vi "trunc_voltages.vi"(5 "Max":dbl, 7 "Min":dbl, 10 "transmissions[r=wl, c=v]":dbl[][](array[numeric]), 11 "voltages":dbl[](array[numeric])) -> (1 "trunc voltages":dbl[](array[numeric]), 2 "Min":dbl, 3 "Max":dbl, 4 "trunc transmissions[r=wl, c=v]":dbl[][](array[numeric]))   [LabVIEW 2019]
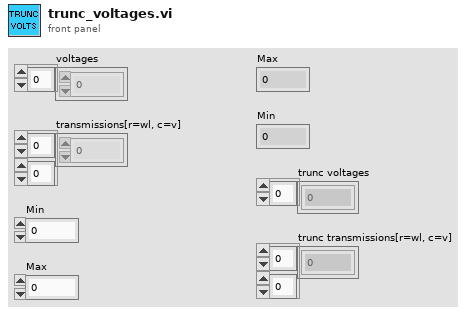
[diagram p1: front panel]
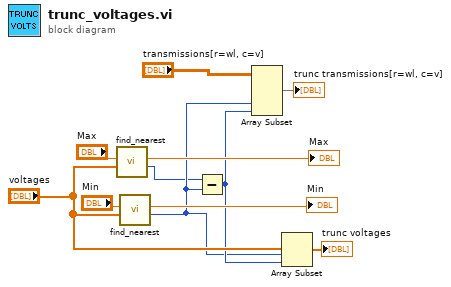
[diagram p0: block diagram]
diagram:
  n1 = call "find_nearest.vi"("Sorted Array (<)"="voltages", "Key"="Max") -> ("Nearest index"=w1:i32, "Nearest"=→"Max":dbl)  [unwired: 6 in, 2 out]
  n2 = call "find_nearest.vi"("Sorted Array (<)"="voltages", "Key"="Min") -> ("Nearest index"=w2:i32, "Nearest"=→"Min":dbl)  [unwired: 6 in, 2 out]
  n3 = Subtract(x=w1, y=w2) -> (x-y=w3:i32)
  n4 = Array Subset(array="transmissions[r=wl, c=v]", index (col)=w2, length (col)=w3) -> (→"trunc transmissions[r=wl, c=v]":dbl[][])  [unwired: 2 in]
  n5 = Array Subset(array="voltages", index=w2, length=w3) -> (→"trunc voltages":dbl[])
